vi "LogLoop.vi"(8 "Error In":errorcluster, 10 "Data Structures":T1, 11 "Action Queues":T2) -> (0 "Error Out":errorcluster)   [LabVIEW 2012]
uses:
  ActionQueues.ctl
  UIActionQueueElement.ctl
  UIAction.ctl
  HardwareActionQueueElement.ctl
  HardwareAction.ctl
  HeaterActionQueueElement.ctl
  HeaterAction.ctl
  MFCActionQueueElement.ctl
  MFCAction.ctl
  LogActionQueueElement.ctl
  LogAction.ctl
  DataStructures.ctl
  HardwareDisplayData.ctl
  HardwareLogData.ctl
  HeaterConfigurationGlobalAction.ctl
  MFCConfigurationGlobalAction.ctl
  <vilib>/Utility/error.llb/DialogType.ctl
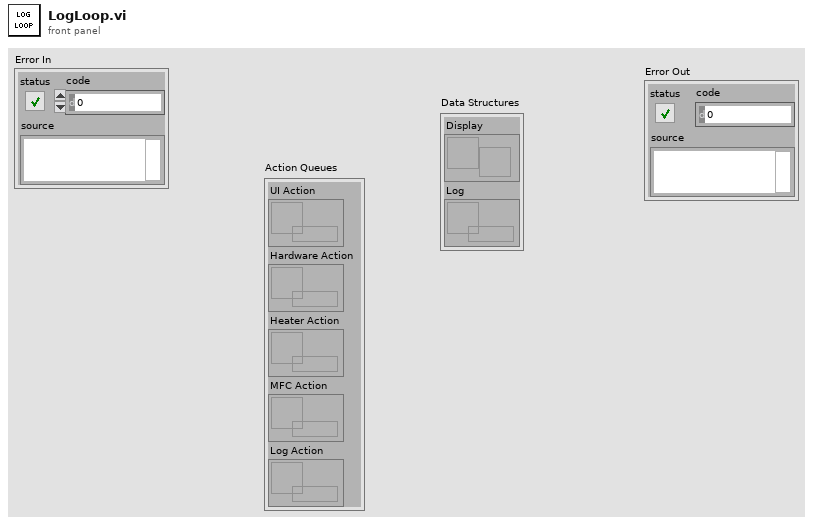
[diagram p1: front panel]
types:
  T1 = typedef "DataStructures.ctl" = cluster{"Display":refnum<notifier>, "Log":refnum<queue>}
  T2 = typedef "ActionQueues.ctl" = cluster{"UI Action":refnum<queue>, "Hardware Action":refnum<queue>, "Heater Action":refnum<queue>, "MFC Action":refnum<queue>, "Log Action":refnum<queue>}
  T3 = typedef "LogActionQueueElement.ctl" = cluster{"Action":T4, "Data":variant}
  T4 = typedef "LogAction.ctl" = enum16{"Initialize", "Start", "Log", "Stop", "Error", "Shutdown"}
  T5 = typedef "MFCConfigurationGlobalAction.ctl" = enum16{"Get", "Set", "Reset"}
  T6 = typedef "HeaterConfigurationGlobalAction.ctl" = enum16{"Get", "Set", "Reset"}
  T7 = typedef "HardwareLogData.ctl" = cluster{"Timestamp":timestamp, "Data":T8}
  T8 = typedef "HardwareDisplayData.ctl" = cluster{"Heater":dbl, "MFC":dbl}
  T9 = typedef "MFCConfiguration.ctl" = cluster{"COM Port":u32, "Timeout (msec)":u32, "Setpoint":dbl, "Valve State":T10, "Gas":T11, "Units":T12, "Serial Number":string, "Firmware Version":string}
  T10 = typedef "Sierra-M100.lvlib/ValveState.ctl" = enum16{"Automatic", "Closed", "Purge"}
  T11 = typedef "Sierra-M100.lvlib/Gas.ctl" = enum16{"Air", "Argon", "CO2", "CO", "Helium", "Hydrogen", "Methane", "Nitrogen", "Nitrous Oxide", "Oxygen"}
  T12 = typedef "Sierra-M100.lvlib/Units.ctl" = enum16{"scc/s", "scc/m", "scc/H", "Ncc/s", "Ncc/m", "Ncc/H", "SCF/s", "SCF/m", "SCF/H", "NM3/s", "NM3/m", "NM3/H", "SM3/s", "SM3/m", "SM3/H", "sl/s", "sl/m", "sl/H", "NL/s", "NL/m", "Nl/H", "g/s", "g/m", "g/H", "kg/s", "kg/m", "kg/H", "lb/s", "lb/m", "lb/H"}
  T13 = typedef "HeaterConfiguration.ctl" = cluster{"COM Port":u8, "Setpoint":dbl, "Standby?":bool}
  T14 = typedef "DialogType.ctl" = u16
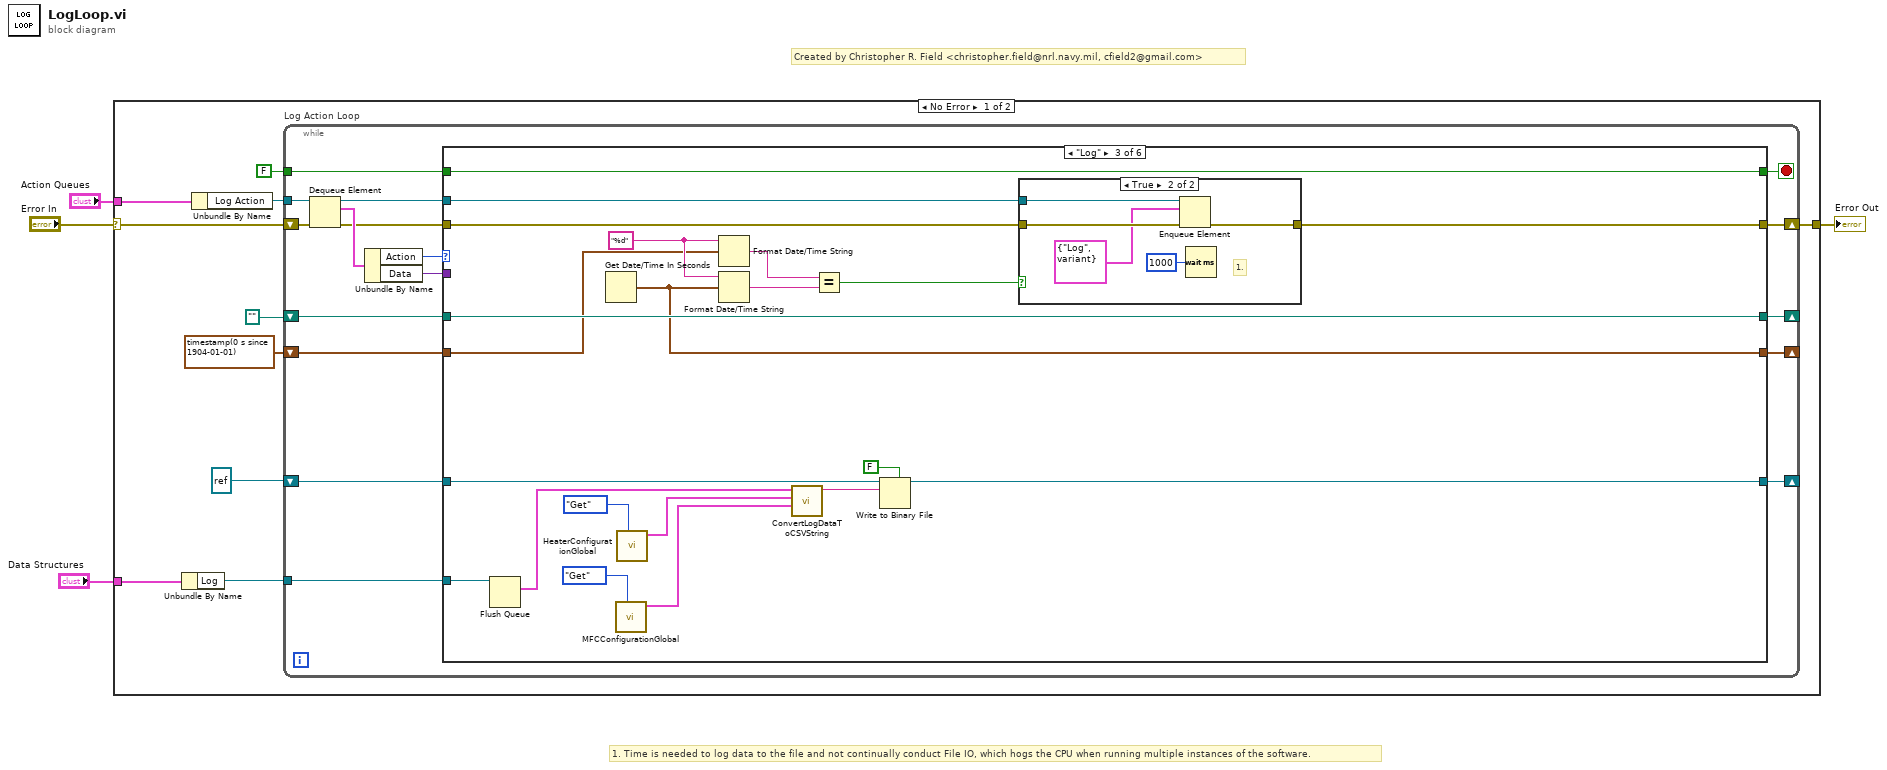
[diagram p0: block diagram]
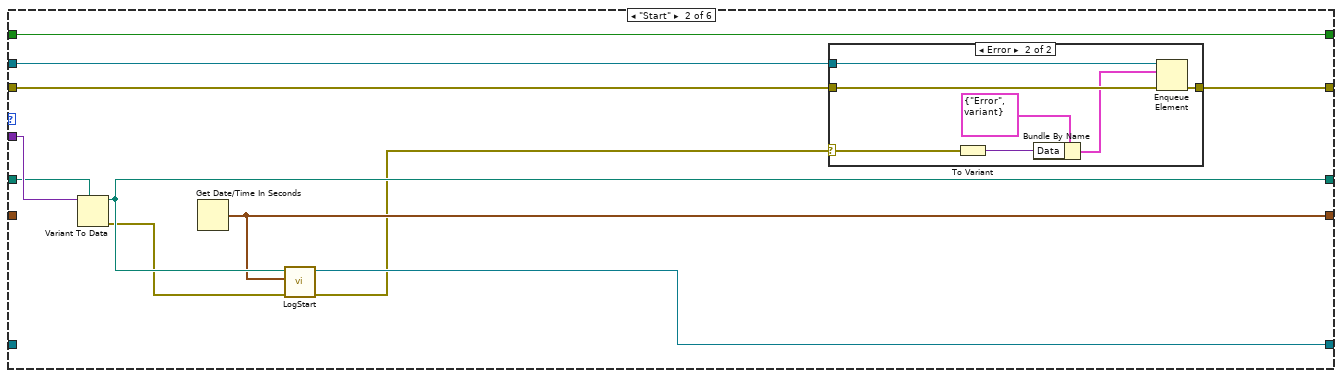
[diagram p3: hidden frame]
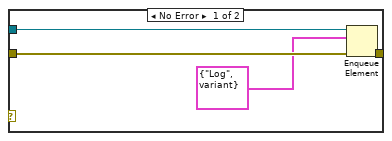
[diagram p4: hidden frame]
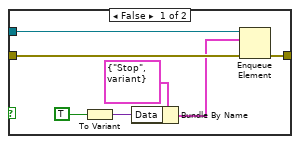
[diagram p5: hidden frame]
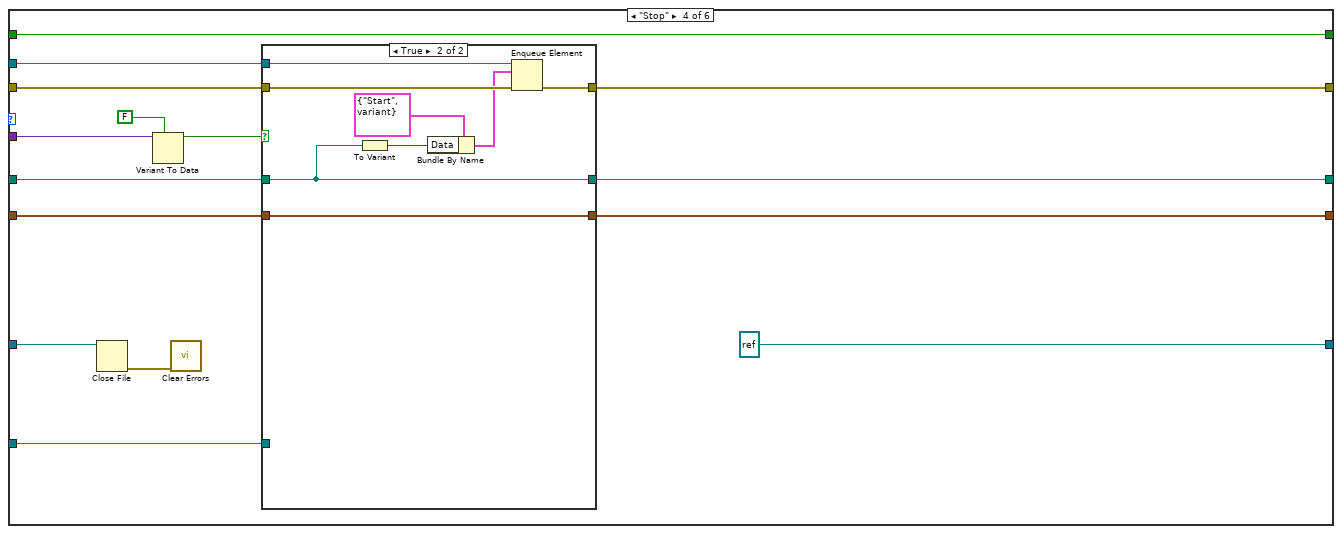
[diagram p6: hidden frame]
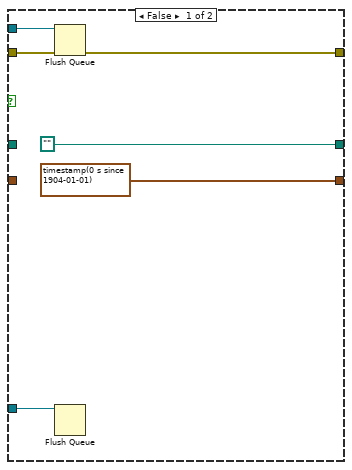
[diagram p7: hidden frame]
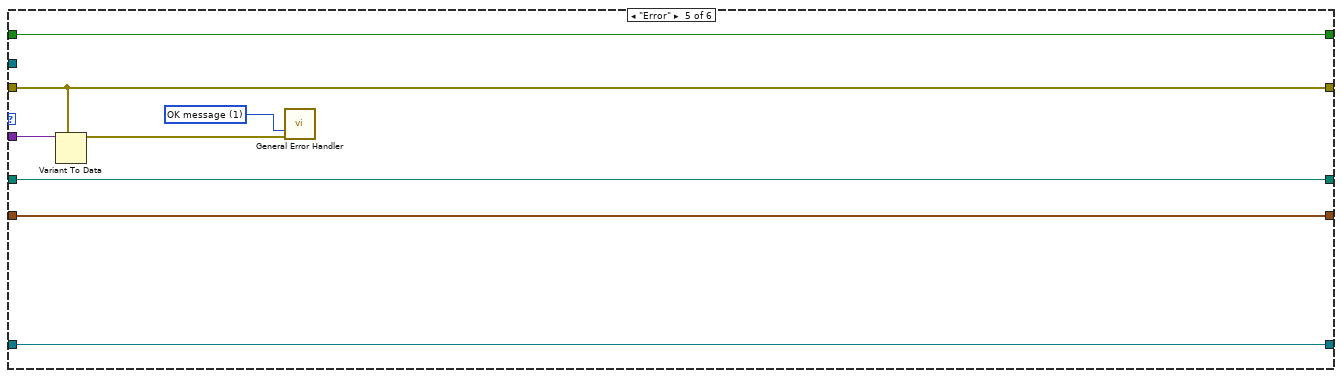
[diagram p8: hidden frame]
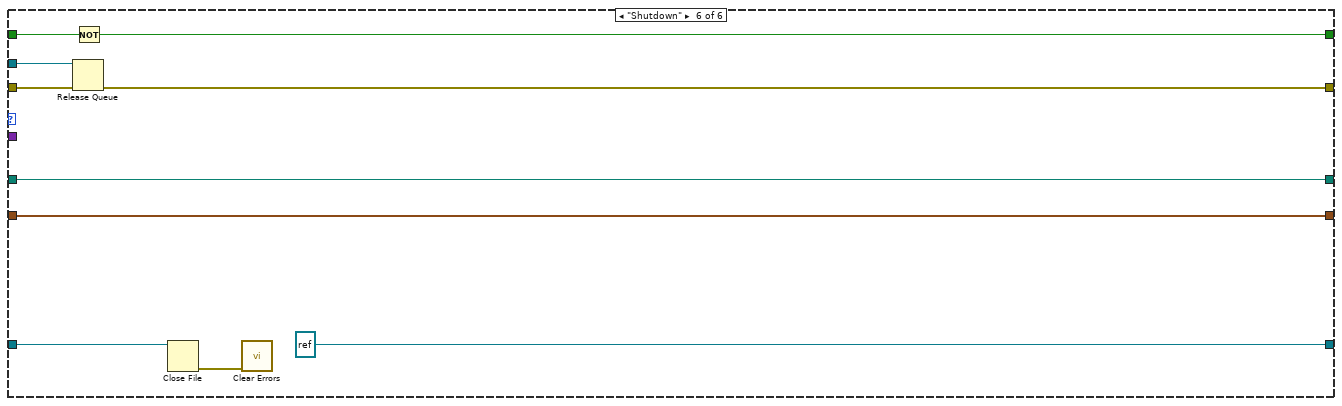
[diagram p9: hidden frame]
diagram:
  # "1. Time is needed to log data to the file and not continually conduct File IO, which hogs the CPU when running multiple instances of the software."
  # "Created by Christopher R. Field <christopher.field@nrl.navy.mil, cfield2@gmail.com>"
  n1 = case shown="No Error" "Error In" {
    selector: "Error In" -> [w14 w139]
    tunnel: [w5 w139] -> w3
    tunnel: "Action Queues" -> [w8 _]
    tunnel: "Data Structures" -> [w7 _]
    frame No Error {
      n2 = Unbundle By Name(w7) -> ("Log"=w6:refnum<queue>)
      n3 = Unbundle By Name(w8) -> ("Log Action"=w9:refnum<queue>)
      n4 = while "Log Action Loop" {
        tunnel: FALSE -> [w25]
        shift-right: [w23] -> w5
        shift-left: w14 -> [w31]
        shift-right: [w21] -> _
        shift-left: path "" -> [w22]
        shift-right: [w20] -> _
        shift-left: refnum<file> refnum ("refnum out") -> [w19]
        shift-right: [w18] -> _
        shift-left: timestamp(0 s since 1904-01-01) ("seconds since 1Jan1904") -> [w17]
        tunnel: w9 -> [w16]
        tunnel: w6 -> [w15]
        stop <- w24 stop-if-true
        n5 = Dequeue Element(queue=w16, error in (no error)=w31) -> (queue out=w26:refnum<queue>, element=w30:T3, error out=w27:errorcluster)  [unwired: 1 in, 1 out]
        n6 = Unbundle By Name(w30) -> ("Action"=w29:T4, "Data"=w28:variant)
        n7 = case shown="\"Log\"" w29 {
          tunnel: w28 -> [_ w43 _ w104 w124 _]
          tunnel: w27 -> [w35 w45 w67 w101 w123 w135]
          tunnel: w26 -> [_ w46 w66 w102 _ w136]
          tunnel: w25 -> [w36 w47 w79 w106 w128 w138]
          tunnel: [w36 w47 w79 w106 w128 w137] -> w24
          tunnel: [w35 w44 w65 w100 w123 w134] -> w23
          tunnel: w22 -> [w33 w42 w74 w97 w127 w133]
          tunnel: [w33 w41 w74 w96 w127 w133] -> w21
          tunnel: [w32 w38 w75 refnum<file> refnum ("refnum out") w125 refnum<file> refnum ("refnum out")] -> w20
          tunnel: w19 -> [w32 _ w77 w99 w125 w130]
          tunnel: [w34 w39 w69 w94 w126 w132] -> w18
          tunnel: w17 -> [w34 _ w70 w95 w126 w132]
          tunnel: w15 -> [_ _ w64 w92 _ _]
          frame "Initialize", Default {
          }
          frame "Start" {
            n8 = Variant To Data(type=w42, Variant=w43) -> (data=w41:path, error out=w40:errorcluster)  [unwired: 1 in]
            n9 = Get Date/Time In Seconds() -> (seconds since 1Jan1904=w39:timestamp)
            n10 = call "LogStart.vi"("Error In"=w40, "Start Time"=w39, "Base Log Path"=w41) -> ("Error Out"=w37:errorcluster, "Log Out"=w38:refnum<file>)  [unwired: 7 in]
            n11 = case shown="Error" w37 {
              selector: w37 -> [_ w53]
              tunnel: w46 -> [w51 w58]
              tunnel: w45 -> [w50 w57]
              tunnel: [w48 w56] -> w44
              frame No Error {
                n12 = Enqueue Element(queue=w51, element=T3 {"Action"=enum."Log", "Data"=variant}, error in (no error)=w50) -> (error out=w48:errorcluster)  [unwired: 1 in, 2 out]
              }
              frame Error {
                n13 = To Variant(anything=w53) -> (Variant=w54:variant)
                n14 = Bundle By Name(cluster=T3 {"Action"=enum."Error", "Data"=variant} ("element"), "Data"=w54) -> (w52:T3)
                n15 = Enqueue Element(queue=w58, element=w52, error in (no error)=w57) -> (error out=w56:errorcluster)  [unwired: 1 in, 2 out]
              }
            }
          }
          frame "Log" {
            w73 = "%d" ("time format string (%c)")
            n16 = Flush Queue(queue=w64) -> (remaining elements=w63:T7[])  [unwired: 1 in, 2 out]
            n17 = Get Date/Time In Seconds() -> (seconds since 1Jan1904=w69:timestamp)
            n18 = call "MFCConfigurationGlobal.vi"("Action"=MFCConfigurationGlobalAction."Get") -> ("Value Out"=w59:T9)  [unwired: 10 in]
            n19 = call "HeaterConfigurationGlobal.vi"("Action"=HeaterConfigurationGlobalAction."Get") -> ("Value Out"=w60:T13)  [unwired: 10 in]
            n20 = Format Date/Time String(time format string (%c)=w73, seconds (now)=w70) -> (date/time string=w72:string)  [unwired: 1 in]
            n21 = Format Date/Time String(time format string (%c)=w73, seconds (now)=w69) -> (date/time string=w71:string)  [unwired: 1 in]
            n22 = call "ConvertLogDataToCSVString.vi"("MFC Configuration"=w59, "Heater Configuration"=w60, "Log Data"=w63) -> ("CSV String"=w78:string)  [unwired: 8 in]
            n23 = Equal?(x=w72, y=w71) -> (x = y?=w68:bool)
            n24 = Write to Binary File(file (use dialog)=w77, data=w78, 5:FALSE ("prepend array or string size? (T)")) -> (refnum out=w75:refnum<file>)  [unwired: 3 in, 2 out]
            n25 = case shown="True" w68 {
              tunnel: w67 -> [w85 w90]
              tunnel: w66 -> [w86 w91]
              tunnel: [w84 w89] -> w65
              frame False {
                n26 = To Variant(anything=TRUE) -> (Variant=w82:variant)
                n27 = Bundle By Name(cluster=T3 {"Action"=enum."Stop", "Data"=variant} ("element"), "Data"=w82) -> (w80:T3)
                n28 = Enqueue Element(queue=w86, element=w80, error in (no error)=w85) -> (error out=w84:errorcluster)  [unwired: 1 in, 2 out]
              }
              frame True {
                # "1."
                n29 = Enqueue Element(queue=w91, element=T3 {"Action"=enum."Log", "Data"=variant}, error in (no error)=w90) -> (error out=w89:errorcluster)  [unwired: 1 in, 2 out]
                n30 = Wait (ms)(milliseconds to wait=u32 1000) -> ()  [unwired: 1 out]
              }
            }
          }
          frame "Stop" {
            n31 = Close File(refnum=w99) -> (error out=w93:errorcluster)  [unwired: 1 in, 1 out]
            n32 = Variant To Data(type=FALSE, Variant=w104) -> (data=w103:bool)  [unwired: 1 in, 1 out]
            n33 = call <vilib>:"Clear Errors.vi"("error in (no error)"=w93) -> ()  [unwired: 6 in, 1 out]
            n34 = case shown="True" w103 {
              tunnel: w102 -> [w112 w120]
              tunnel: w101 -> [w111 w119]
              tunnel: [w110 w118] -> w100
              tunnel: w97 -> [_ w114]
              tunnel: [path "" w114] -> w96
              tunnel: w95 -> [_ w113]
              tunnel: [timestamp(0 s since 1904-01-01) ("seconds since 1Jan1904") w113] -> w94
              tunnel: w92 -> [w107 _]
              frame False {
                n35 = Flush Queue(queue=w112, error in (no error)=w111) -> (error out=w110:errorcluster)  [unwired: 2 out]
                n36 = Flush Queue(queue=w107) -> ()  [unwired: 1 in, 3 out]
              }
              frame True {
                n37 = To Variant(anything=w114) -> (Variant=w116:variant)
                n38 = Bundle By Name(cluster=T3 {"Action"=enum."Start", "Data"=variant} ("element"), "Data"=w116) -> (w115:T3)
                n39 = Enqueue Element(queue=w120, element=w115, error in (no error)=w119) -> (error out=w118:errorcluster)  [unwired: 1 in, 2 out]
              }
            }
          }
          frame "Error" {
            w121 = T14 1 items=["no dialog", "OK message", "continue or stop message", "OK message + warnings", "continue/stop + warnings"] ("type of dialog (OK msg:1)")
            n40 = Variant To Data(type=w123, Variant=w124) -> (data=w122:errorcluster)  [unwired: 1 in, 1 out]
            n41 = call <vilib>:"General Error Handler.vi"("type of dialog (OK msg:1)"=w121, "error in (no error)"=w122) -> ()  [unwired: 9 in, 5 out]
          }
          frame "Shutdown" {
            n42 = Release Queue(queue=w136, error in (no error)=w135) -> (error out=w134:errorcluster)  [unwired: 1 in, 2 out]
            n43 = Not(x=w138) -> (.not. x?=w137:bool)
            n44 = Close File(refnum=w130) -> (error out=w131:errorcluster)  [unwired: 1 in, 1 out]
            n45 = call <vilib>:"Clear Errors.vi"("error in (no error)"=w131) -> ()  [unwired: 6 in, 1 out]
          }
        }
      }
    }
    frame Error {
    }
  }
  "Error Out" <- w3
